vi "AG34980A_Configure_Data_Format.vi"(0 "VISA resource name":refnum<visa-resource-name>, 5 "Alarm Enable (F:Off)":bool, 7 "Channel Enable (F:Off)":bool, 9 "Unit Enable (F:Off)":bool, 11 "error in (no error)":errorcluster, 12 "Time Enable (F:Off)":bool, 13 "Time Type (1:Relative)":enum16{"Absolute", "Relative"}(ring)=enum."Relative") -> (4 "VISA resource name out":refnum<visa-resource-name>, 15 "error out":errorcluster)   [LabVIEW 2022 SP3, in "DMM_Keysight_34980A.lvlib" / "DMM_Keysight_34980A.lvclass"]
doc: "This VI allows you to control the format of data that is returned from measurements. You can optionally choose to include channel number information, alarm information, time information, and measurement units information."
uses:
  DMM_Keysight_34980A.lvclass
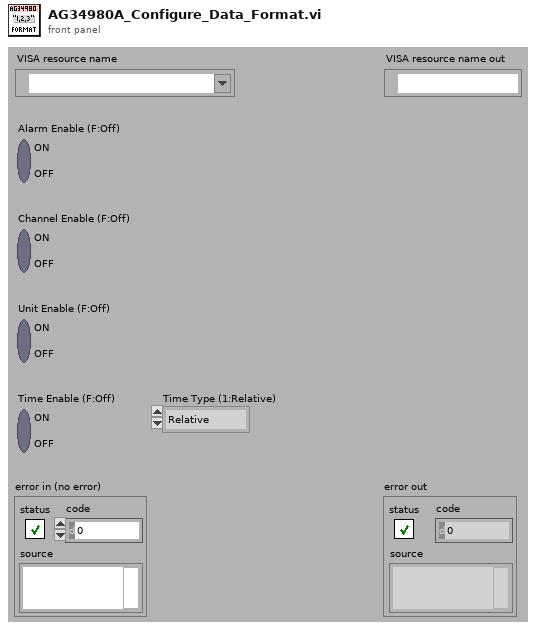
[diagram p1: front panel]
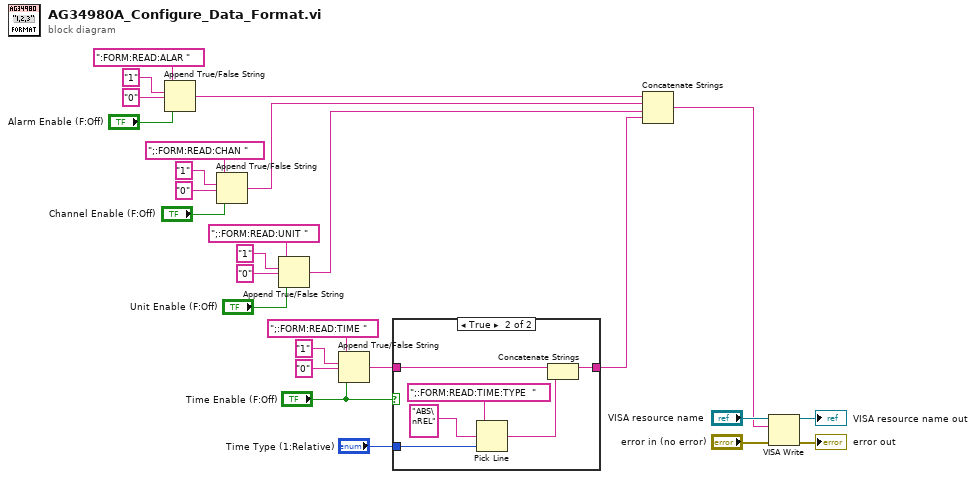
[diagram p0: block diagram]
diagram:
  n1 = Append True/False String(1:"Alarm Enable (F:Off)", 2:"0" ("false string"), 3:"1" ("true string"), 4:":FORM:READ:ALAR ") -> (0:w9:string)
  n2 = Append True/False String(1:"Channel Enable (F:Off)", 2:"0" ("false string"), 3:"1" ("true string"), 4:";:FORM:READ:CHAN ") -> (0:w8:string)
  n3 = Append True/False String(1:"Unit Enable (F:Off)", 2:"0" ("false string"), 3:"1" ("true string"), 4:";:FORM:READ:UNIT ") -> (0:w6:string)
  n4 = Append True/False String(1:"Time Enable (F:Off)", 2:"0" ("false string"), 3:"1" ("true string"), 4:";:FORM:READ:TIME ") -> (0:w3:string)
  n5 = case shown="True" "Time Enable (F:Off)" {
    tunnel: "Time Type (1:Relative)" -> [_ w33]
    tunnel: w3 -> [w28 w32]
    tunnel: [w28 w29] -> w2
    frame False {
    }
    frame True {
      n6 = Pick Line(string ("")=";:FORM:READ:TIME:TYPE  ", multi-line string="ABS\nREL", line index=w33) -> (output string=w31:string)
      n7 = Concatenate Strings(w32, w31) -> (w29:string)
    }
  }
  n8 = Concatenate Strings(w9, w8, w6, w2) -> (w1:string)
  n9 = VISA Write(VISA resource name="VISA resource name", write buffer=w1, error in (no error)="error in (no error)") -> (VISA resource name out=→"VISA resource name out":refnum<visa-resource-name>, error out=→"error out":errorcluster)  [unwired: 1 out]
